vi "differential-drive-pose-est-test.vi"(8 "error in (no error)":errorcluster) -> (0 "error out":errorcluster, 3 "Test Passed":bool)   [LabVIEW 2019]
uses:
  <vilib>/Rock Robotics/SystemInterfaces/NetworkCommunication/NetComm_UsageReport_report.vi
  <vilib>/Rock Robotics/WPI/ThirdParty/JAS_Junk/TrajLib/MatBuilder_Create.vi
  <vilib>/Rock Robotics/WPI/ThirdParty/JAS_Junk/TrajLib/MatrixHelper_CoerceSize.vi
  <vilib>/Rock Robotics/WPI/ThirdParty/JAS_Junk/TrajLib/Rotation_RotateBy.vi
  <vilib>/Rock Robotics/WPI/ThirdParty/JAS_Junk/TrajLib/Util_CalcDist.vi
  <vilib>/Rock Robotics/WPI/ThirdParty/JAS_Junk/TrajLib/Rotation_CreateXY.vi
  <vilib>/Rock Robotics/WPI/ThirdParty/JAS_Junk/TrajLib/Util_LibraryGlobals.vi
  <vilib>/Analysis/1siggen.llb/Gaussian White Noise.vi
  <vilib>/Rock Robotics/WPI/ThirdParty/JAS_Junk/TrajLib/Trajectory_Library.lvlib
  <vilib>/ptbypt/NI_PtbyPt.lvlib
panel:
  out "Add Vision Error":bool
  out "BenchProcessing \nTimer Per Pass":dbl
  out "BenchTotalTime":dbl
  out "BenchTotalPasses":dbl
  out "MaxErrPassed":bool
  out "MeanPassed":bool
  out "ErrorSumNormalized":dbl
  out "Error Sum":dbl
  out "Max Error":dbl
  out "Using Vision":bool
  in  "UseVIsion":bool=TRUE
  out "VIsionUpdates":i32
  out "TotalTImeSecs":dbl
  out "Position Graph":cluster{dbl[], dbl[]}[](graph)
  out "PoesEstCreateErr":bool
  # "< 0.055"
  # "< 0.035"
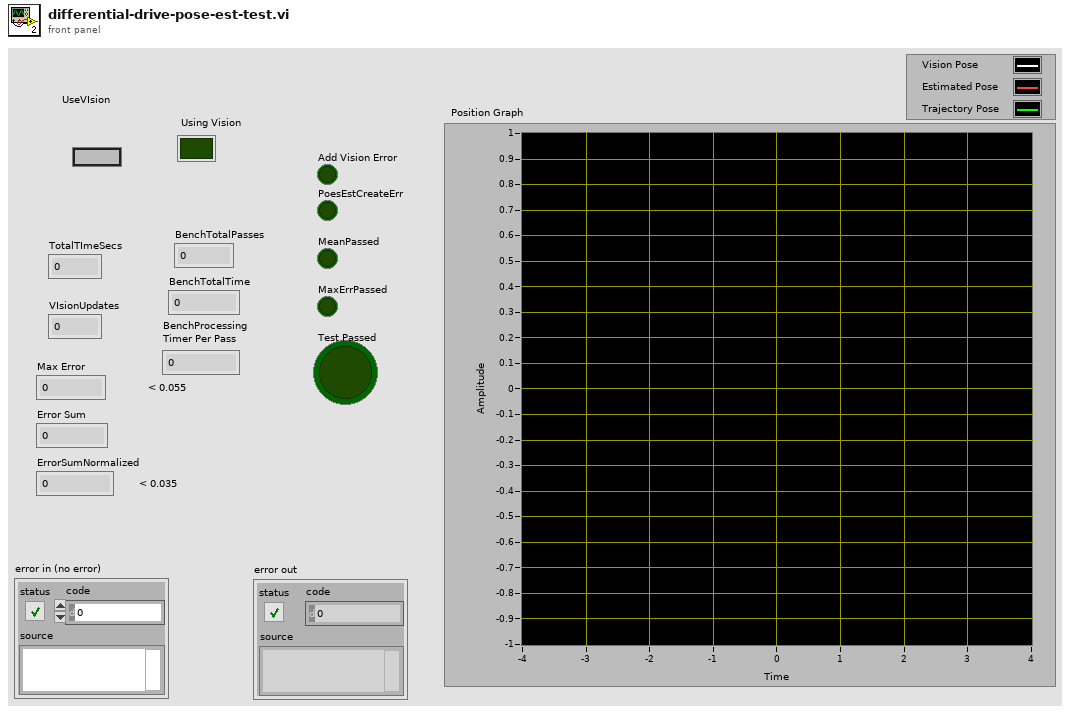
[diagram p1: front panel]
types:
  T1 = typedef "Trajectory_Library.lvlib/ROTATION2D.ctl" = cluster{"VALUE":dbl, "COS":dbl, "SIN":dbl}
  T2 = typedef "Trajectory_Library.lvlib/POSE2D.ctl" = cluster{"TRANSLATION":T3, "ROTATION":T1}
  T3 = typedef "Trajectory_Library.lvlib/TRANSLATION2D.ctl" = cluster{"X":dbl, "Y":dbl}
  T4 = typedef "NI_Matrix.lvlib/RealMatrix.ctl" = dbl[][]
  T5 = typedef "Trajectory_Library.lvlib/DIFF_DRIVE_KINEMATICS.ctl" = cluster{"TrackWidth_Meters":dbl}
  T6 = typedef "Trajectory_Library.lvlib/TRAJ_CONFIG.ctl" = cluster{"MaxVelocity":dbl, "Max Acceleration":dbl, "StartVelocity":dbl, "End Velocity":dbl, "Reversed":bool, "DiffDrKineConstntDefined":bool, "CentAcellConstntDefined":bool, "DiffDrVoltConstntDefined":bool, "DIFF_DRIVE_KINE_CONSTRAINT":T7, "CENTRIPETAL_ACCEL_CONSTRAINT":T8, "SwerveDrKineConstntDefined":bool, "SWERVE_DRIVE_KINE_CONSTRAINT":T9, "DIFF_DRIVE_VOLTAGE_CONSTRAINT":T11, "MECANUM_DRIVE_KINE_CONSTRAINT":T13, "MecanumDrKineConstntDefined":bool}
  T7 = typedef "Trajectory_Library.lvlib/TRAJ_CONSTRAINT_DIIF_DRIVE_KINEMATICS.ctl" = cluster{"Max Speed (M/S)":dbl, "DIFF_DRIVE_KINEMATICS":T5, "Max Accel (M/S2)":dbl}
  T8 = typedef "Trajectory_Library.lvlib/TRAJ_CONSTRAINT_CENTRIPETAL_ACCEL.ctl" = cluster{"Max Cent Accel":dbl}
  T9 = typedef "Trajectory_Library.lvlib/TRAJ_CONSTRAINT_SWERVE_DRIVE_KINEMATICS.ctl" = cluster{"Max Speed (M/S)":dbl, "SwerveKinematics":T10}
  T10 = typedef "Trajectory_Library.lvlib/SWERVE_DRIVE_KINEMATICS.ctl" = cluster{"NumModules":i32, "InverseKinematics":T4, "ForwardKinematics":T4, "Modules":T3[], "PrevCoR":T3}
  T11 = typedef "Trajectory_Library.lvlib/TRAJ_CONSTRAINT_DIIF_DRIVE_VOLTAGE.ctl" = cluster{"Max Voltage":dbl, "DIFF_DRIVE_KINEMATICS":T5, "SIMPLE_MOTOR_FF":T12}
  T12 = typedef "Trajectory_Library.lvlib/SIMPLE_MOTOR_FF.ctl" = cluster{"Ks":dbl, "Kv":dbl, "Ka":dbl}
  T13 = typedef "Trajectory_Library.lvlib/TRAJ_CONSTRAINT_MECA_DRIVE_KINEMATICS.ctl" = cluster{"Max Speed (M/S)":dbl, "MECA_DRIVE_KINEMATICS":T14}
  T14 = typedef "Trajectory_Library.lvlib/MECA_DRIVE_KINEMATICS.ctl" = cluster{"FrontLeft":T3, "FrontRight":T3, "RearLeft":T3, "RearRight":T3, "InverseKinematics":T4, "ForwardKinematics":T4, "PrevCoR":T3}
  T15 = typedef "Trajectory_Library.lvlib/DIFF_DRIVE_POSE_EST.ctl" = cluster{"M_VisionContR":T4, "m_nominal_dT":dbl, "m_PrevTime_Sec":dbl, "m_GyroOffset":T1, "m_PrevAngle":T1, "StartLeftEnc_M":dbl, "StartRightEnc_M":dbl, "m_Observer":T16, "m_latencyCompensator":T19}
  T16 = typedef "Trajectory_Library.lvlib/UNSCENTED_KALMAN_FILTER.ctl" = cluster{"m_P":T4, "m_xHat":T4, "States":i32, "Outputs":i32, "m_ContR":T4, "m_ContQ":T4, "m_SigmasF":T4, "m_dT_Sec":dbl, "MERWE_SCALED_SIGMA_PTS":T17, "meanFuncX":T18, "meanFuncY":T18, "residualFuncX":T18, "residualFuncY":T18, "addFuncX":T18, "addFuncXExtra":variant, "residualFuncYExtra":variant, "residualFuncXExtra":variant, "MeanFuncYExtra":variant, "MeanFuncXExtra":variant, "Inputs":i32}
  T17 = typedef "Trajectory_Library.lvlib/MERWE_SCALED_SIGMA_PTS.ctl" = cluster{"m_Wm":T4, "States":i32, "Alpha":dbl, "m_Wc":T4, "Kappa":i32}
  T18 = typedef "Trajectory_Library.lvlib/CALLBACK_FUNC_TYPE.ctl" = refnum<vi>
  T19 = typedef "Trajectory_Library.lvlib/KALMAN_FILTER_LATENCY_COMP.ctl" = cluster{"m_pastObserverSnapshots ":T20[]}
  T20 = typedef "Trajectory_Library.lvlib/OBSERVER_SNAP_LIST_ITEM.ctl" = cluster{"TimeStamp":dbl, "OBSERVER_SNAPSHOT":T21}
  T21 = typedef "Trajectory_Library.lvlib/OBSERVER_SNAPSHOT.ctl" = cluster{"ErrorCoVariance":T4, "xHat":T4, "LocalMeasurements":T4, "Inputs":T4}
  T22 = typedef "Trajectory_Library.lvlib/TRAJECTORY.ctl" = cluster{"TotalTImeSecs":dbl, "States":T23[]}
  T23 = typedef "Trajectory_Library.lvlib/TRAJ_STATE.ctl" = cluster{"TimeSeconds":dbl, "Velocity":dbl, "Acceleration":dbl, "POSE":T2, "Curvature":dbl}
  T24 = typedef "Trajectory_Library.lvlib/CHASSIS_SPEEDS.ctl" = cluster{"vX":dbl, "vY":dbl, "vOmega":dbl}
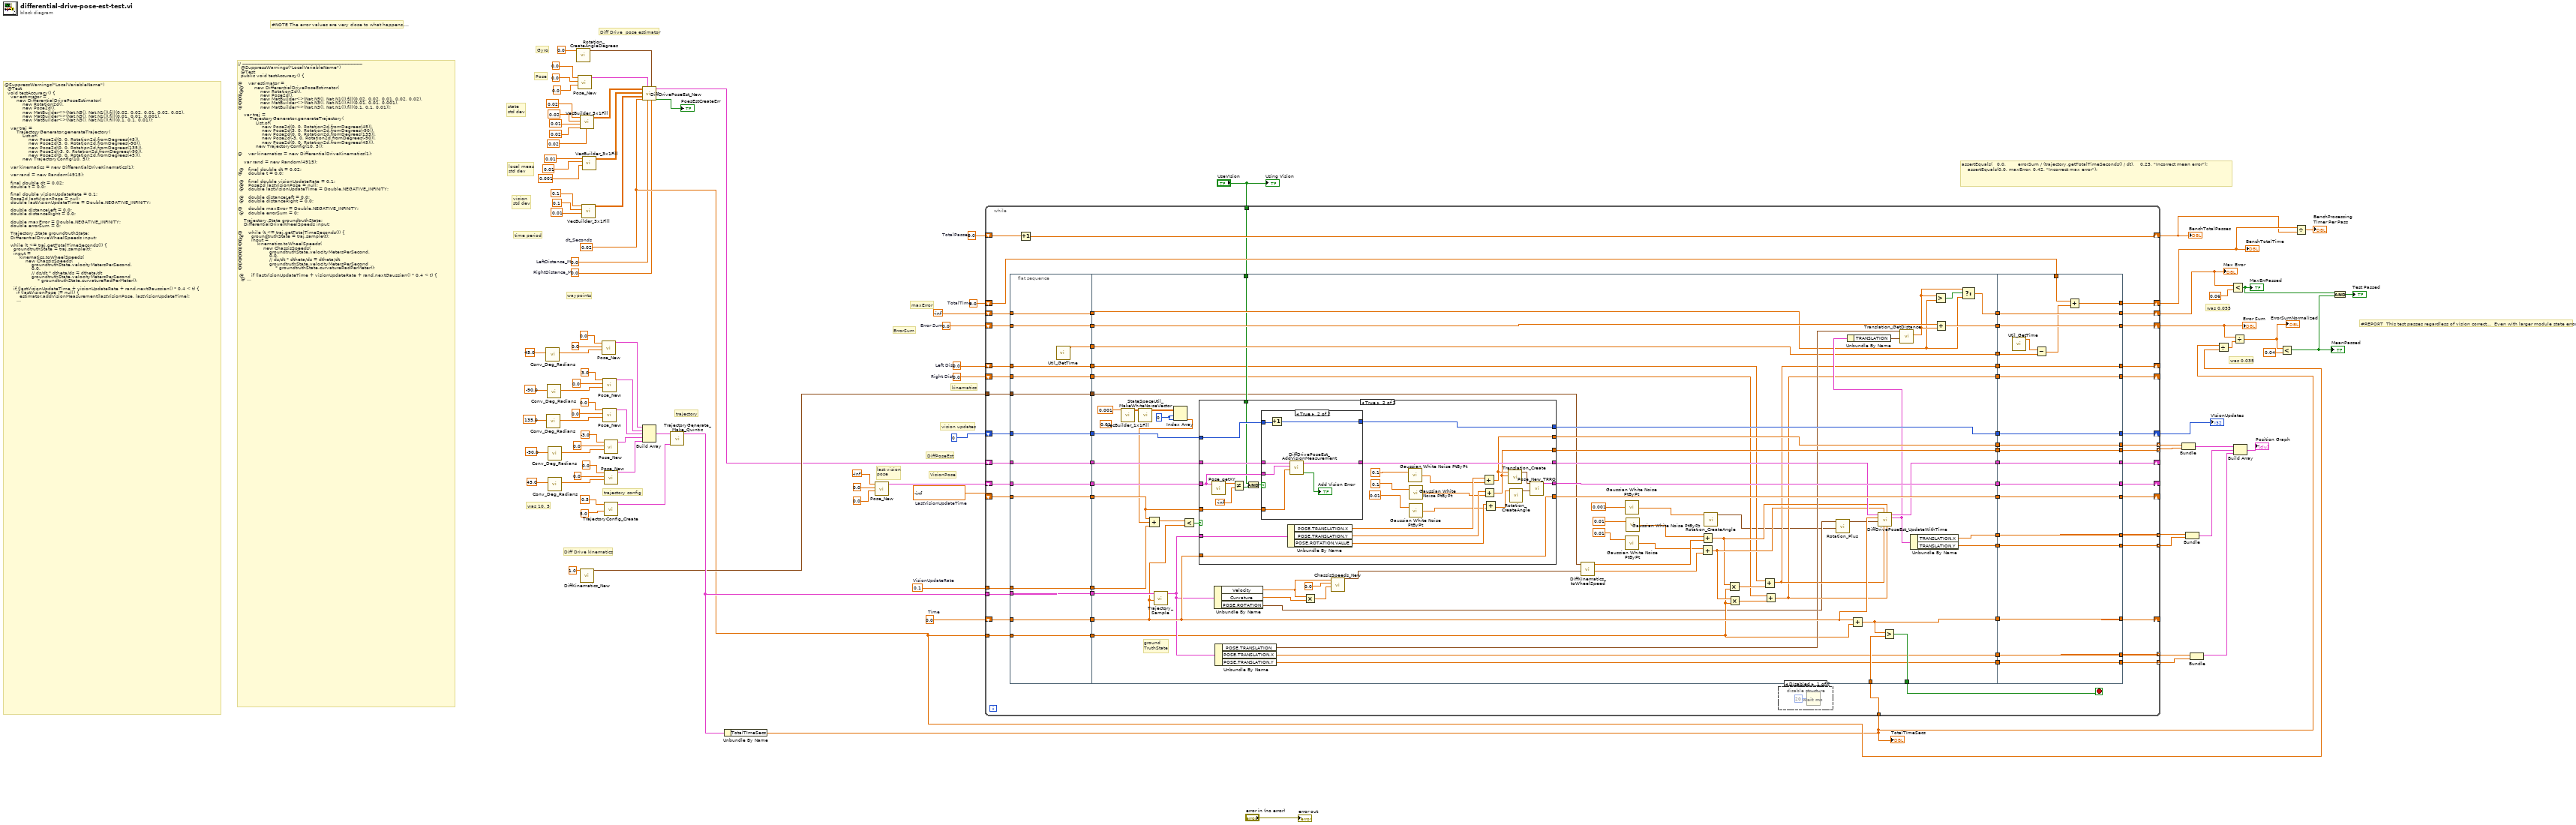
[diagram p0: block diagram]
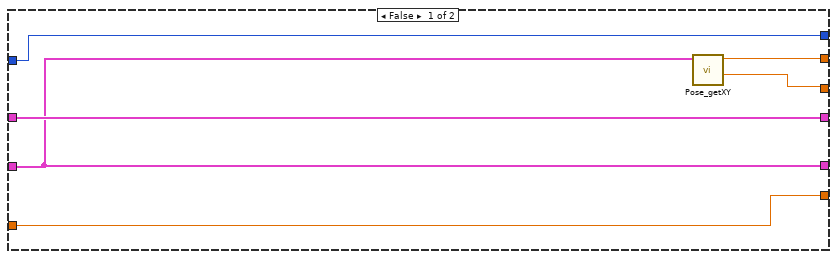
[diagram p3: hidden frame]
diagram:
  w2 = 0.0  # Right Dist
  w3 = 0.0  # Left Dist
  w10 = 0.0  # RightDistance_M
  w11 = 0.0  # LeftDistance_M
  w16 = 0.0  # TotalPasses
  w17 = 0.0  # TotalTime
  w29 = 0.0  # Error Sum
  w48 = 0.1  # VisionUpdateRate
  w49 = -inf  # LastVisionUpdateTime
  w51 = 0.0  # Time
  w27 = 0.02  # dt_Seconds
  # "was 10, 5"
  # "@SuppressWarnings(\"LocalVariableName\")\n  @Test\n  void testAccuracy() {\n    var estimator =\n        new DifferentialDrivePoseEstimator(\n            new Rotation2d(),\n            new Pose2d(),\n            new MatBuilder<>(Nat.N5(), Nat.N1()).fill(0.02, 0.02, 0.01, 0.02, 0.02),\n            new MatBuilder<>(Nat.N3(), Nat.N1()).fill(0.01, 0.01, 0.001),\n            new MatBuilder<>(Nat.N3(), Nat.N1()).fill(0.1, 0.1, 0.01));\n\n    var traj =\n        TrajectoryGenerator.generateTrajectory(\n            List.of(\n                new Pose2d(0, 0, Rotation2d.fromDegrees(45)),\n                new Pose2d(3, 0, Rotation2d.fromDegrees(-90)),\n                new Pose2d(0, 0, Rotation2d.fromDegrees(135)),\n                new Pose2d(-3, 0, Rotation2d.fromDegrees(-90)),\n                new Pose2d(0, 0, Rotation2d.fromDegrees(45))),\n            new TrajectoryConfig(10, 5));\n\n    var kinematics = new DifferentialDriveKinematics(1);\n\n    var rand = new Random(4915);\n\n    final double dt = 0.02;\n    double t = 0.0;\n\n    final double visionUpdateRate = 0.1;\n    Pose2d lastVisionPose = null;\n    double lastVisionUpdateTime = Double.NEGATIVE_INFINITY;\n\n    double distanceLeft = 0.0;\n    double distanceRight = 0.0;\n\n    double maxError = Double.NEGATIVE_INFINITY;\n    double errorSum = 0;\n\n    Trajectory.State groundtruthState;\n    DifferentialDriveWheelSpeeds input;\n\n    while (t <= traj.getTotalTimeSeconds()) {\n      groundtruthState = traj.sample(t);\n      input =\n          kinematics.toWheelSpeeds(\n              new ChassisSpeeds(\n                  groundtruthState.velocityMetersPerSecond,\n                  0.0,\n                  // ds/dt * dtheta/ds = dtheta/dt\n                  groundtruthState.velocityMetersPerSecond\n                      * groundtruthState.curvatureRadPerMeter));\n\n      if (lastVisionUpdateTime + visionUpdateRate + rand.nextGaussian() * 0.4 < t) {\n        if (lastVisionPose != null) {\n          estimator.addVisionMeasurement(lastVisionPose, lastVisionUpdateTime);\n        }\n        var groundPose = groundtruthState.poseMeters;\n        lastVisionPose =\n            new Pose2d(\n                new Translation2d(\n                    groundPose.getTranslation().getX() + rand.nextGaussian() * 0.1,\n                    groundPose.getTranslation().getY() + rand.nextGaussian() * 0.1),\n                new Rotation2d(rand.nextGaussian() * 0.01).plus(groundPose.getRotation()));\n        lastVisionUpdateTime = t;\n      }\n\n      input.leftMetersPerSecond += rand.nextGaussian() * 0.01;\n      input.rightMetersPerSecond += rand.nextGaussian() * 0.01;\n\n      distanceLeft += input.leftMetersPerSecond * dt;\n      distanceRight += input.rightMetersPerSecond * dt;\n\n      var rotNoise = new Rotation2d(rand.nextGaussian() * 0.001);\n\n      var xHat =\n          estimator.updateWithTime(\n              t,\n              groundtruthState.poseMeters.getRotation().plus(rotNoise),\n              input,\n              distanceLeft,\n              distanceRight);\n\n      double error =\n          groundtruthState.poseMeters.getTranslation().getDistance(xHat.getTranslation());\n      if (error > maxError) {\n        maxError = error;\n      }\n      errorSum += error;\n\n      t += dt;\n    }\n\n    assertEquals(0.0, errorSum / (traj.getTotalTimeSeconds() / dt), 0.035, \"Incorrect mean error\");\n    assertEquals(0.0, maxError, 0.055, \"Incorrect max error\");\n  }\n}"
  # "was 0.055"
  # "was 0.035"
  # "#NOTE The error values are very close to what happens...."
  # "// --------------------------------------------------------------------------------\n  @SuppressWarnings(\"LocalVariableName\")\n  @Test\n  public void testAccuracy() {\n\n@    var estimator =\n @       new DifferentialDrivePoseEstimator(\n @           new Rotation2d(),\n@            new Pose2d(),\n@            new MatBuilder<>(Nat.N5(), Nat.N1()).fill(0.02, 0.02, 0.01, 0.02, 0.02),\n@            new MatBuilder<>(Nat.N3(), Nat.N1()).fill(0.01, 0.01, 0.001),\n@            new MatBuilder<>(Nat.N3(), Nat.N1()).fill(0.1, 0.1, 0.01));\n\n    var traj =\n        TrajectoryGenerator.generateTrajectory(\n            List.of(\n                new Pose2d(0, 0, Rotation2d.fromDegrees(45)),\n                new Pose2d(3, 0, Rotation2d.fromDegrees(-90)),\n                new Pose2d(0, 0, Rotation2d.fromDegrees(135)),\n                new Pose2d(-3, 0, Rotation2d.fromDegrees(-90)),\n                new Pose2d(0, 0, Rotation2d.fromDegrees(45))),\n            new TrajectoryConfig(10, 5));\n\n@    var kinematics = new DifferentialDriveKinematics(1);\n\n    var rand = new Random(4915);\n\n @   final double dt = 0.02;\n@    double t = 0.0;\n\n @   final double visionUpdateRate = 0.1;\n @   Pose2d lastVisionPose = null;\n @   double lastVisionUpdateTime = Double.NEGATIVE_INFINITY;\n\n @   double distanceLeft = 0.0;\n @   double distanceRight = 0.0;\n\n@    double maxError = Double.NEGATIVE_INFINITY;\n @   double errorSum = 0;\n\n    Trajectory.State groundtruthState;\n    DifferentialDriveWheelSpeeds input;\n\n@    while (t <= traj.getTotalTimeSeconds()) {\n @     groundtruthState = traj.sample(t);\n@      input =\n@          kinematics.toWheelSpeeds(\n@              new ChassisSpeeds(\n@                  groundtruthState.velocityMetersPerSecond,\n@                  0.0,\n@                  // ds/dt * dtheta/ds = dtheta/dt\n@                  groundtruthState.velocityMetersPerSecond\n@                      * groundtruthState.curvatureRadPerMeter));\n\n @     if (lastVisionUpdateTime + visionUpdateRate + rand.nextGaussian() * 0.4 < t) {\n  @      if (lastVisionPose != null) {\n  @        estimator.addVisionMeasurement(lastVisionPose, lastVisionUpdateTime);\n @       }\n @       var groundPose = groundtruthState.poseMeters;\n @       lastVisionPose =\n  @          new Pose2d(\n  @              new Translation2d(\n  @                  groundPose.getTranslation().getX() + rand.nextGaussian() * 0.1,\n  @                  groundPose.getTranslation().getY() + rand.nextGaussian() * 0.1),\n  @              new Rotation2d(rand.nextGaussian() * 0.01).plus(groundPose.getRotation()));\n  @      lastVisionUpdateTime = t;\n  @    }\n\n@      input.leftMetersPerSecond += rand.nextGaussian() * 0.01;\n @     input.rightMetersPerSecond += rand.nextGaussian() * 0.01;\n\n@      distanceLeft += input.leftMetersPerSecond * dt;\n@      distanceRight += input.rightMetersPerSecond * dt;\n\n @     var rotNoise = new Rotation2d(rand.nextGaussian() * 0.001);\n\n @     var xHat =\n @         estimator.updateWithTime(\n @             t,\n  @            groundtruthState.poseMeters.getRotation().plus(rotNoise),\n  @            input,\n @             distanceLeft,\n @             distanceRight);\n\n @     double error =\n @         groundtruthState.poseMeters.getTranslation().getDistance(xHat.getTranslation());\n  @    if (error > maxError) {\n  @      maxError = error;\n  @    }\n  @    errorSum += error;\n\n  @    t += dt;\n  @  }   // END OF WHILE LOOP\n\n    assertEquals(0.0, errorSum / (traj.getTotalTimeSeconds() / dt), 0.035, \"Incorrect mean error\");\n    assertEquals(0.0, maxError, 0.055, \"Incorrect max error\");\n  }\n}"
  # "#REPORT  This test passes regardless of vision correct...  Even with larger module state errors"
  # "assertEquals(   0.0,        errorSum / (trajectory.getTotalTimeSeconds() / dt),    0.25, \"Incorrect mean error\");\n    assertEquals(0.0, maxError, 0.42, \"Incorrect max error\");"
  # "ErrorSum"
  # "maxError"
  # "vision updates"
  # "kinematics"
  # "DiffPoseEst"
  # "VisionPose"
  # "last vision\npose"
  # "time period"
  # "vision \nstd dev"
  # "local meas\nstd dev"
  # "state\nstd dev"
  # "Pose"
  # "Gyro"
  # "Diff Drive  pose estimator"
  # "Diff Drive kinematics"
  # "trajectory config"
  # "trajectory"
  # "waypoints"
  n1 = call <vilib>:"Conv_Deg_Radians.vi"("Degress"=45.0 ("Heading")) -> ("Radians"=w74:dbl)  [unwired: 10 in]
  n2 = call <vilib>:"Conv_Deg_Radians.vi"("Degress"=135.0 ("Heading")) -> ("Radians"=w82:dbl)  [unwired: 10 in]
  n3 = call <vilib>:"Conv_Deg_Radians.vi"("Degress"=-90.0 ("Heading")) -> ("Radians"=w78:dbl)  [unwired: 10 in]
  n4 = call <vilib>:"Conv_Deg_Radians.vi"("Degress"=-90.0 ("Heading")) -> ("Radians"=w86:dbl)  [unwired: 10 in]
  n5 = call <vilib>:"Conv_Deg_Radians.vi"("Degress"=45.0 ("Heading")) -> ("Radians"=w90:dbl)  [unwired: 10 in]
  n6 = call <vilib>:"Rotation_CreateAngleDegrees.vi"("Angle_Degrees"=0.0) -> ("ROTATION"=w68:T1)  [unwired: 10 in]
  n7 = call <vilib>:"Pose_New.vi"("Heading"=0.0, "Y"=0.0, "X"=0.0) -> ("out POSe"=w66:T2)  [unwired: 8 in]
  n8 = call <vilib>:"VecBuilder_5x1Fill.vi"("R4"=0.02, "R3"=0.02, "R2"=0.01 ("element"), "R1"=0.02 ("element"), "R0"=0.02 ("element")) -> ("output matrix"=w58:T4)  [unwired: 6 in]
  n9 = call <vilib>:"DiffKinematics_New.vi"("TrackWidth_Meters"=1.0) -> ("DIFF_DRIVE_KINEMATICS"=w42:T5)  [unwired: 10 in]
  n10 = call <vilib>:"VecBuilder_3x1Fill.vi"("R2"=0.01 ("element"), "R1"=0.1 ("element"), "R0"=0.1 ("element")) -> ("output matrix"=w53:T4)  [unwired: 8 in]
  n11 = call <vilib>:"VecBuilder_3x1Fill.vi"("R2"=0.001, "R1"=0.01, "R0"=0.01 ("element")) -> ("output matrix"=w57:T4)  [unwired: 8 in]
  n12 = call <vilib>:"Pose_New.vi"("Heading"=w74, "Y"=0.0, "X"=0.0) -> ("out POSe"=w73:T2)  [unwired: 8 in]
  n13 = call <vilib>:"Pose_New.vi"("Heading"=w82, "Y"=0.0, "X"=0.0) -> ("out POSe"=w70:T2)  [unwired: 8 in]
  n14 = call <vilib>:"Pose_New.vi"("Heading"=w78, "Y"=0.0, "X"=3.0) -> ("out POSe"=w71:T2)  [unwired: 8 in]
  n15 = call <vilib>:"Pose_New.vi"("Heading"=w86, "Y"=0.0, "X"=-3.0) -> ("out POSe"=w69:T2)  [unwired: 8 in]
  n16 = call <vilib>:"Pose_New.vi"("Heading"=w90, "Y"=0.0, "X"=0.0) -> ("out POSe"=w95:T2)  [unwired: 8 in]
  n17 = call <vilib>:"TrajectoryConfig_Create.vi"("MaxAcceleration"=5.0, "MaxVelocity"=0.5) -> ("TRAJECTORY_CONFIG"=w92:T6)  [unwired: 9 in]
  n18 = call <vilib>:"DiffDrivePoseEst_New.vi"("RightDistance_M"=w10, "gyroAngle"=w68, "LeftDistance_M"=w11, "InitialPose"=w66, "dt_Seconds"=w27, "VisionMeasurementStdDevs"=w53, "LocalMeasurementStdDevs"=w57, "StateStdDevs"=w58) -> ("Error"=→"PoesEstCreateErr":bool, "DiffDrivePoseEstimate"=w9:T15)  [unwired: 2 in]
  n19 = Build Array(w73, w71, w70, w69, w95) -> (w93:T2[])
  n20 = call <vilib>:"TrajectoryGenerate_Make_Quintic.vi"("traj_config"=w92, "waypointPOSE"=w93) -> ("TRAJECTORY"=w50:T22)  [unwired: 8 in, 1 out]
  n21 = Unbundle By Name(w50) -> ("TotalTImeSecs"=w20:dbl)
  "TotalTImeSecs" <- w20
  n22 = call <vilib>:"Pose_New.vi"("Heading"=0.0, "Y"=0.0, "X"=-inf) -> ("out POSe"=w44:T2)  [unwired: 8 in]
  n23 = while {
    tunnel: w27 -> [w162]
    shift-right: [w161] -> _
    shift-left: w51 -> [w149]
    tunnel: w50 -> [w159]
    tunnel: w20 -> [w160]
    shift-right: [w153] -> _
    shift-left: w49 -> [w155]
    tunnel: w48 -> [w158]
    shift-right: [w154] -> _
    shift-left: w44 -> [w157]
    shift-right: [w106] -> _
    shift-left: w9 -> [w156]
    tunnel: [w152] -> w43 mode=indexing
    tunnel: [w151] -> w41 mode=indexing
    tunnel: [w148] -> w40 mode=indexing
    tunnel: [w147] -> w39 mode=indexing
    shift-right: [w145] -> w34
    shift-left: 0 -> [w146]
    tunnel: [w144] -> w33 mode=indexing
    tunnel: [w143] -> w32 mode=indexing
    shift-right: [w140] -> w25
    shift-left: -inf -> [w139]
    shift-right: [w141] -> w28
    shift-left: w29 -> [w142]
    shift-right: [w111] -> w15
    shift-left: w17 -> [w110]
    shift-right: [w108] -> w14
    shift-left: w16 -> [w109]
    tunnel: "UseVIsion" -> [w107]
    shift-right: [w101] -> _
    shift-left: w3 -> [w104]
    shift-right: [w99] -> _
    shift-left: w2 -> [w102]
    tunnel: w42 -> [w150]
    stop <- w138 stop-if-true
    n24 = flat-sequence {
      tunnel: w139 -> [w167]
      tunnel: w142 -> [w168]
      tunnel: w146 -> [w169]
      tunnel: w149 -> [w170]
      tunnel: w150 -> [w171]
      tunnel: w155 -> [w172]
      tunnel: w156 -> [w173]
      tunnel: w157 -> [w174]
      tunnel: w158 -> [w175]
      tunnel: w159 -> [w176]
      tunnel: w162 -> [w177]
      tunnel: [w177] -> w137
      tunnel: [w176] -> w136
      tunnel: [w175] -> w135
      tunnel: [w174] -> w134
      tunnel: [w173] -> w133
      tunnel: [w172] -> w132
      tunnel: [w171] -> w131
      tunnel: [w170] -> w130
      tunnel: [w169] -> w129
      tunnel: [w168] -> w128
      tunnel: [w167] -> w127
      tunnel: [w166] -> w113
      tunnel: [w165] -> w105
      tunnel: w104 -> [w165]
      tunnel: [w164] -> w103
      tunnel: w102 -> [w164]
      tunnel: [w243] -> w138
      tunnel: w160 -> [w241]
      tunnel: w137 -> [w201]
      tunnel: w136 -> [w240]
      tunnel: w135 -> [w184]
      tunnel: w134 -> [w237]
      tunnel: w133 -> [w236]
      tunnel: w132 -> [w235]
      tunnel: w131 -> [w204]
      tunnel: w130 -> [w226]
      tunnel: w129 -> [w222]
      tunnel: w128 -> [w214]
      tunnel: w127 -> [w209]
      tunnel: [w242] -> w126
      tunnel: [w234] -> w125
      tunnel: [w233] -> w124
      tunnel: [w232] -> w123
      tunnel: [w231] -> w122
      tunnel: [w225] -> w121
      tunnel: [w224] -> w120
      tunnel: [w223] -> w119
      tunnel: [w221] -> w118
      tunnel: [w219] -> w117
      tunnel: [w218] -> w116
      tunnel: [w213] -> w115
      tunnel: [w210] -> w114
      tunnel: w113 -> [w208]
      tunnel: [w208] -> w112
      tunnel: w107 -> [w207]
      tunnel: w105 -> [w196]
      tunnel: w103 -> [w195]
      tunnel: [w194] -> w100
      tunnel: [w193] -> w98
      tunnel: [w294] -> w140
      tunnel: [w295] -> w141
      tunnel: [w296] -> w143
      tunnel: [w297] -> w144
      tunnel: [w298] -> w145
      tunnel: [w299] -> w147
      tunnel: [w300] -> w148
      tunnel: [w301] -> w106
      tunnel: [w302] -> w151
      tunnel: [w303] -> w152
      tunnel: [w304] -> w153
      tunnel: [w305] -> w154
      tunnel: [w306] -> w161
      tunnel: w126 -> [w306]
      tunnel: w125 -> [w305]
      tunnel: w124 -> [w304]
      tunnel: w123 -> [w303]
      tunnel: w122 -> [w302]
      tunnel: w121 -> [w301]
      tunnel: w120 -> [w300]
      tunnel: w119 -> [w299]
      tunnel: w118 -> [w298]
      tunnel: w117 -> [w297]
      tunnel: w116 -> [w296]
      tunnel: w115 -> [w295]
      tunnel: w114 -> [w294]
      tunnel: w112 -> [w292]
      tunnel: [w291] -> w111
      tunnel: w110 -> [w289]
      tunnel: [w288] -> w101
      tunnel: w100 -> [w288]
      tunnel: [w287] -> w99
      tunnel: w98 -> [w287]
      frame #0 {
        n25 = call <vilib>:"Util_GetTime.vi"() -> ("FPGA_Time_Seconds"=w166:dbl)  [unwired: 10 in, 1 out]
      }
      frame #1 {
        (unwired) 0.01 ("R0")
        w186 = 0 ("index (col)")
        # "ground\nTruthState"
        n26 = call <vilib>:"VecBuilder_1x1Fill.vi"("R0_C0"=0.001 ("R0")) -> ("output matrix"=w189:T4)  [unwired: 10 in]
        n27 = call <vilib>:"StateSpaceUtil_MakeWhiteNoiseVector.vi"("StdDevs"=w189) -> ("WhiteNoise"=w187:T4)  [unwired: 9 in, 1 out]
        n28 = call <vilib>:"Trajectory_Sample.vi"("Time"=w226, "InputTRAJECTORY"=w240) -> ("OutputTRAJ_STATE"=w220:T23)  [unwired: 9 in]
        n29 = Index Array(array=w187, index (row)=w186, index (col)=w186) -> (element=w185:dbl)
        n30 = Compound Arithmetic op=ADD(w235, w185, w184) -> (w238:dbl)
        n31 = Less?(x=w238, y=w226) -> (x < y?=w239:bool)
        n32 = case shown="True" w239 {
          tunnel: w237 -> [w247 w274]
          tunnel: w236 -> [w249 w275]
          tunnel: [w249 w273] -> w206
          tunnel: w235 -> [w248 w272]
          tunnel: w220 -> [_ w269]
          tunnel: [w247 w271] -> w234
          tunnel: w226 -> [_ w266]
          tunnel: [w248 w266] -> w233
          tunnel: [w246 w265] -> w232
          tunnel: [w245 w264] -> w231
          tunnel: w222 -> [w244 w263]
          tunnel: [w244 w262] -> w221
          tunnel: w207 -> [_ w259]
          frame False {
            n33 = call <vilib>:"Pose_getXY.vi"("in POSE"=w247) -> ("Y"=w245:dbl, "X"=w246:dbl)  [unwired: 9 in]
          }
          frame True {
            n34 = call <vilib>:"Pose_getXY.vi"("in POSE"=w274) -> ("X"=w277:dbl)  [unwired: 9 in, 1 out]
            n35 = Not Equal?(x=w277, y=-inf) -> (x != y?=w260:bool)
            n36 = And(x=w259, y=w260) -> (x .and. y?=w261:bool)
            n37 = case shown="True" w261 {
              tunnel: w275 -> [w279 w282]
              tunnel: w274 -> [_ w286]
              tunnel: [w279 w280] -> w273
              tunnel: w272 -> [_ w285]
              tunnel: w263 -> [w278 w284]
              tunnel: [w278 w283] -> w262
              frame False {
              }
              frame True {
                n38 = Increment(x=w284) -> (x+1=w283:i32)
                n39 = call <vilib>:"DiffDrivePoseEst_AddVisionMeasurement.vi"("TImeStamp_Seconds"=w285, "visionRobotPose"=w286, "in DiffDrivePoseEstimate"=w282) -> ("Error"=→"Add Vision Error":bool, "Out DiffDrivePoseEstimate"=w280:T15)  [unwired: 7 in]
              }
            }
            n40 = Unbundle By Name(w269) -> ("POSE.TRANSLATION.X"=w258:dbl, "POSE.TRANSLATION.Y"=w257:dbl, "POSE.ROTATION.VALUE"=w256:dbl)
            n41 = call <vilib>:"Gaussian White Noise PtByPt.vi"("standard deviation"=0.1 ("R0")) -> ("Gaussian white noise"=w252:dbl)  [unwired: 2 in]
            n42 = call <vilib>:"Gaussian White Noise PtByPt.vi"("standard deviation"=0.01 ("R2")) -> ("Gaussian white noise"=w250:dbl)  [unwired: 2 in]
            n43 = call <vilib>:"Gaussian White Noise PtByPt.vi"("standard deviation"=0.1 ("R1")) -> ("Gaussian white noise"=w251:dbl)  [unwired: 2 in]
            n44 = Add(x=w258, y=w252) -> (x+y=w265:dbl)
            n45 = Add(x=w257, y=w251) -> (x+y=w264:dbl)
            n46 = Add(x=w256, y=w250) -> (x+y=w267:dbl)
            n47 = call <vilib>:"Translation_Create.vi"("Y"=w264, "X"=w265) -> ("TRANSLATION"=w270:T3)  [unwired: 9 in]
            n48 = call <vilib>:"Rotation_CreateAngle.vi"("Angle"=w267) -> ("ROTATION"=w268:T1)  [unwired: 10 in]
            n49 = call <vilib>:"Pose_New_TRRO.vi"("ROTATION"=w268, "TRANSLATION"=w270) -> ("outPOSE"=w271:T2)  [unwired: 9 in]
          }
        }
        n50 = Unbundle By Name(w220) -> ("Velocity"=w228:dbl, "Curvature"=w229:dbl, "POSE.ROTATION"=w191:T1)
        n51 = Unbundle By Name(w220) -> ("POSE.TRANSLATION"=w217:T3, "POSE.TRANSLATION.X"=w218:dbl, "POSE.TRANSLATION.Y"=w219:dbl)
        n52 = Multiply(x=w228, y=w229) -> (x*y=w227:dbl)
        n53 = call <vilib>:"ChassisSpeeds_New.vi"("vAngular"=w227, "vY"=0.0, "vX"=w228) -> ("CHASSIS"=w205:T24)  [unwired: 8 in]
        n54 = call <vilib>:"DiffKinematics_toWheelSpeed.vi"("CHASSIS Speed"=w205, "DIFF_DRIVE_KINEMATICS"=w204) -> ("RightVelocity"=w199:dbl, "LeftVelocity"=w203:dbl)  [unwired: 8 in]
        n55 = call <vilib>:"Gaussian White Noise PtByPt.vi"("standard deviation"=0.001 ("R0")) -> ("Gaussian white noise"=w183:dbl)  [unwired: 2 in]
        n56 = call <vilib>:"Gaussian White Noise PtByPt.vi"("standard deviation"=0.01 ("R1")) -> ("Gaussian white noise"=w181:dbl)  [unwired: 2 in]
        n57 = call <vilib>:"Gaussian White Noise PtByPt.vi"("standard deviation"=0.01 ("R0")) -> ("Gaussian white noise"=w182:dbl)  [unwired: 2 in]
        n58 = Add(x=w181, y=w199) -> (x+y=w202:dbl)
        n59 = Add(x=w182, y=w203) -> (x+y=w200:dbl)
        n60 = call <vilib>:"Rotation_CreateAngle.vi"("Angle"=w183) -> ("ROTATION"=w190:T1)  [unwired: 10 in]
        n61 = Multiply(x=w200, y=w201) -> (x*y=w197:dbl)
        n62 = Multiply(x=w202, y=w201) -> (x*y=w198:dbl)
        n63 = Add(x=w196, y=w197) -> (x+y=w194:dbl)
        n64 = Add(x=w195, y=w198) -> (x+y=w193:dbl)
        n65 = call <vilib>:"Rotation_Plus.vi"("other ROTATION"=w190, "in ROTATION"=w191) -> ("out ROTATION"=w192:T1)  [unwired: 9 in]
        n66 = Add(x=w226, y=w201) -> (x+y=w242:dbl)
        n67 = call <vilib>:"DiffDrivePoseEst_UpdateWithTime.vi"("RightDistance"=w193, "LeftSpeed"=w200, "LeftDistance"=w194, "RightSpeed"=w202, "GyroAngle"=w192, "CurrentTimeSeconds"=w226, "in DiffDrivePoseEstimate"=w206) -> ("Estimated Pose"=w216:T2, "Out DiffDrivePoseEstimate"=w225:T15)  [unwired: 2 in, 1 out]
        n68 = Unbundle By Name(w216) -> ("TRANSLATION"=w215:T3)
        n69 = Greater?(x=w242, y=w241) -> (0:w243:bool)
        n70 = call <vilib>:"Translation_GetDistance.vi"("other Translation"=w215, "In Translation"=w217) -> ("Distance"=w211:dbl)  [unwired: 9 in]
        n71 = Unbundle By Name(w216) -> ("TRANSLATION.X"=w224:dbl, "TRANSLATION.Y"=w223:dbl)
        n72 = Greater?(x=w211, y=w209) -> (0:w212:bool)
        n73 = Add(x=w214, y=w211) -> (x+y=w213:dbl)
        n74 = Select(t=w211, s=w212, f=w209) -> (s? t:f=w210:dbl)
      }
      frame #2 {
        n75 = call <vilib>:"Util_GetTime.vi"() -> ("FPGA_Time_Seconds"=w293:dbl)  [unwired: 10 in, 1 out]
        n76 = Subtract(x=w293, y=w292) -> (x-y=w290:dbl)
        n77 = Add(x=w289, y=w290) -> (x+y=w291:dbl)
      }
    }
    n78 = Increment(x=w109) -> (x+1=w108:dbl)
    n79 = disable-structure shown="Disabled" {
      frame Disabled {
        n80 = Wait (ms)(milliseconds to wait=u32 20) -> ()  [unwired: 1 out]
      }
      frame Enabled {
      }
    }
  }
  "VIsionUpdates" <- w34
  "Max Error" <- w25
  "Error Sum" <- w28
  "BenchTotalPasses" <- w14
  "BenchTotalTime" <- w15
  n81 = Bundle(w43, w41) -> (w38:cluster{dbl[], dbl[]})  [unwired: 1 in]
  n82 = Bundle(w40, w39) -> (w37:cluster{dbl[], dbl[]})  [unwired: 1 in]
  n83 = Bundle(w32, w33) -> (w31:cluster{dbl[], dbl[]})  [unwired: 1 in]
  n84 = Divide(x=w20, y=w27) -> (x/y=w18:dbl)
  n85 = Less?(x=w25, y=0.06) -> (x < y?=w23:bool)
  "MaxErrPassed" <- w23
  n86 = Divide(x=w28, y=w18) -> (x/y=w19:dbl)
  "ErrorSumNormalized" <- w19
  n87 = Build Array(w38, w37, w31) -> (→"Position Graph":cluster{dbl[], dbl[]}[])
  n88 = Less?(x=w19, y=0.04) -> (x < y?=w22:bool)
  "MeanPassed" <- w22
  n89 = Divide(x=w15, y=w14) -> (x/y=→"BenchProcessing \nTimer Per Pass":dbl)
  n90 = And(x=w23, y=w22) -> (x .and. y?=→"Test Passed":bool)
  "Using Vision" <- "UseVIsion"
  "error out" <- "error in (no error)"
